vi "ADO Error Helper.vi"(8 "Overriding error or warning":errorcluster, 9 "source":string, 10 "code":i32, 11 "status":bool) -> (0 "error out":errorcluster)   [LabVIEW 2011]
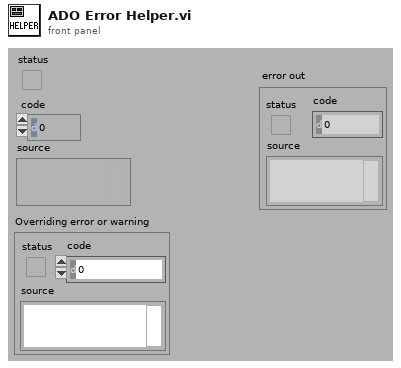
[diagram p1: front panel]
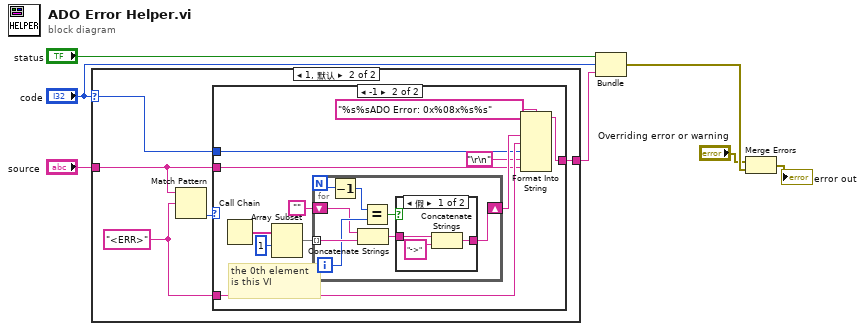
[diagram p0: block diagram]
diagram:
  n1 = case shown="1, 默认" "code" {
    selector: "code" -> [_ w9]
    tunnel: [w8 w13] -> w2
    tunnel: "source" -> [w8 w10]
    frame 0 {
    }
    frame 1, Default {
      w12 = "<ERR>" ("Substring")
      n2 = Match Pattern(string=w10, regular expression=w12) -> (offset past match=w11:i32)  [unwired: 4 out]
      n3 = case shown="-1" w11 {
        tunnel: [w14 w19] -> w13
        tunnel: w10 -> [w14 w16]
        tunnel: w12 -> [_ w20]
        tunnel: w9 -> [_ w17]
        frame 0, Default {
        }
        frame -1 {
          # "the 0th element\nis this VI"
          n4 = Call Chain() -> (call chain=w22:string[])
          n5 = Array Subset(array=w22, index=1 ("Array Index")) -> (w24:string[])  [unwired: 1 in]
          n6 = for {
            N -> [w32]
            tunnel: w24 -> [w33] mode=indexing
            shift-right: [w26] -> w21
            shift-left: "" -> [w27]
            i -> [w30]
            n7 = Decrement(x=w32) -> (x-1=w31:i32)
            n8 = Concatenate Strings(w27, w33) -> (w28:string)
            n9 = Equal?(x=w31, y=w30) -> (x = y?=w29:bool)
            n10 = case shown="假" w29 {
              tunnel: w28 -> [w36 w37]
              tunnel: [w34 w37] -> w26
              frame False {
                n11 = Concatenate Strings(w36, "->" ("Substring")) -> (w34:string)
              }
              frame True {
              }
            }
          }
          n12 = Format Into String(format string="%s%sADO Error: 0x%08x%s%s", w21, w20, w17, "\r\n", w16) -> (resulting string=w19:string)  [unwired: 2 in, 1 out]
        }
      }
    }
  }
  n13 = Bundle("status"="status", "code"="code", "source"=w2) -> (w7:errorcluster)  [unwired: 1 out]
  n14 = Merge Errors("Overriding error or warning", w7) -> (→"error out":errorcluster)
